vi "API test.vi"() -> ()   [LabVIEW 2014, in "Simple Sequencer TBM tests.lvlib"]
uses:
  Simple Sequencer TBM tests.lvlib
  module/configuration/Simple Sequencer TBM configuration.lvclass
  sequencer parent classes/action configuration parent/action configuration.lvclass
  module/configuration/sequence definition.ctl
  <vilib>/NI/TBM Modules/Sequencer/actions/dwell/Dwell Config.lvclass
  <vilib>/NI/TBM Modules/Sequencer/actions/template action/configuration/Template Action Config.lvclass
  module/execution/Simple Sequencer TBM runtime.lvclass
  simple sequencer api/Simple Sequencer API.lvclass
  <vilib>/NI/TBM Modules/Sequencer/actions/dwell/runtime/Dwell.lvclass
  <vilib>/NI/TBM Modules/Sequencer/actions/template action/runtime/Template Action.lvclass
panel:
  out "String":string
  in  "continue location":i32=-1
  in  "sequences":string[](array[string])
  out "error out 2":errorcluster
  out "error out":errorcluster
  out "available sequences":string[](array[string])
  in  "Resume":bool
  in  "Stop Sequence":bool
  in  "Pause Button":bool
  in  "Play Button":bool
  in  "stop":bool
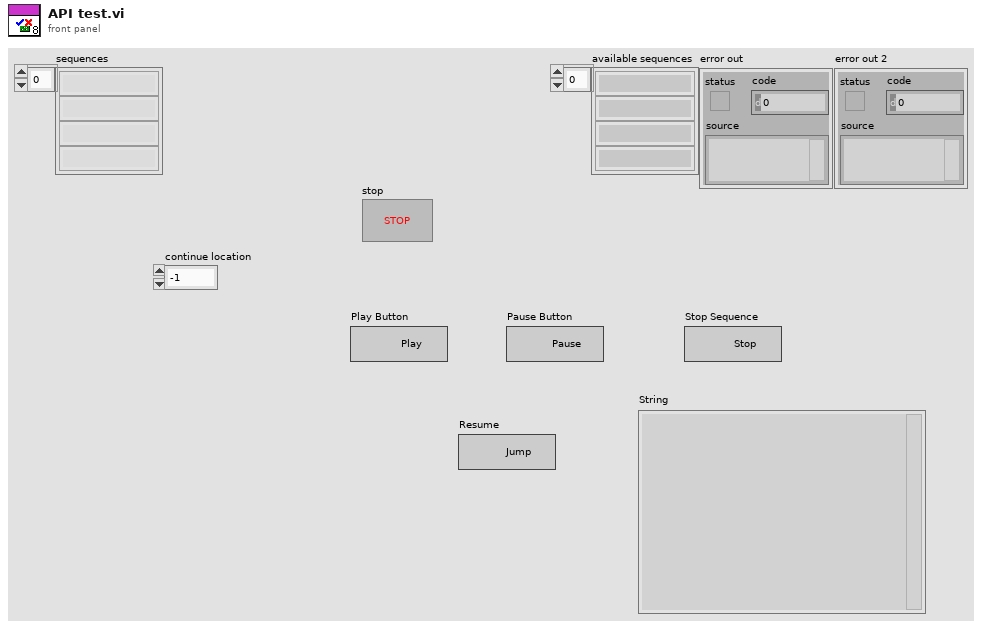
[diagram p1: front panel]
types:
  T1 = typedef "Simple Sequencer TBM configuration.lvclass/sequence definition.ctl" = cluster{"sequence name":string, "action configs":refnum<class "action configuration.lvclass">[]}
  T2 = typedef "TBM channel.lvclass/data tables.ctl" = cluster{"input data":T3, "processing parameter":T3, "processing result":T3, "output data":T3}
  T3 = typedef "tag bus.lvlib/dictionary table pair.ctl" = cluster{"data dictionary":refnum<class "data dictionary.lvclass">, "data table":T4}
  T4 = typedef "tag bus.lvlib/data table.lvlib/data table.ctl" = cluster{"Double":dbl[], "Single":sgl[], "I64":i64[], "I32":i32[], "I16":i16[], "I8":i8[], "U64":u64[], "U32":u32[], "U16":u16[], "U8":u8[], "Boolean":bool[], "String":string[], "Array of Double":cluster{"DBL Array":dbl[]}[], "Array of Single":cluster{"SGL Array":sgl[]}[], "Array of I64":cluster{"I64 Array":i64[]}[], "Array of I32":cluster{"I32 Array":i32[]}[], "Array of I16":cluster{"I16 Array":i16[]}[], "Array of I8":cluster{"I8 Array":i8[]}[], "Array of U64":cluster{"U64 Array":u64[]}[], "Array of U32":cluster{"U32 Array":u32[]}[], "Array of U16":cluster{"U16 Array":u16[]}[], "Array of U8":cluster{"U8 Array":u8[]}[], "Array of Boolean":cluster{"Boolean Array":bool[]}[], "Array of String":cluster{"String Array":string[]}[]}
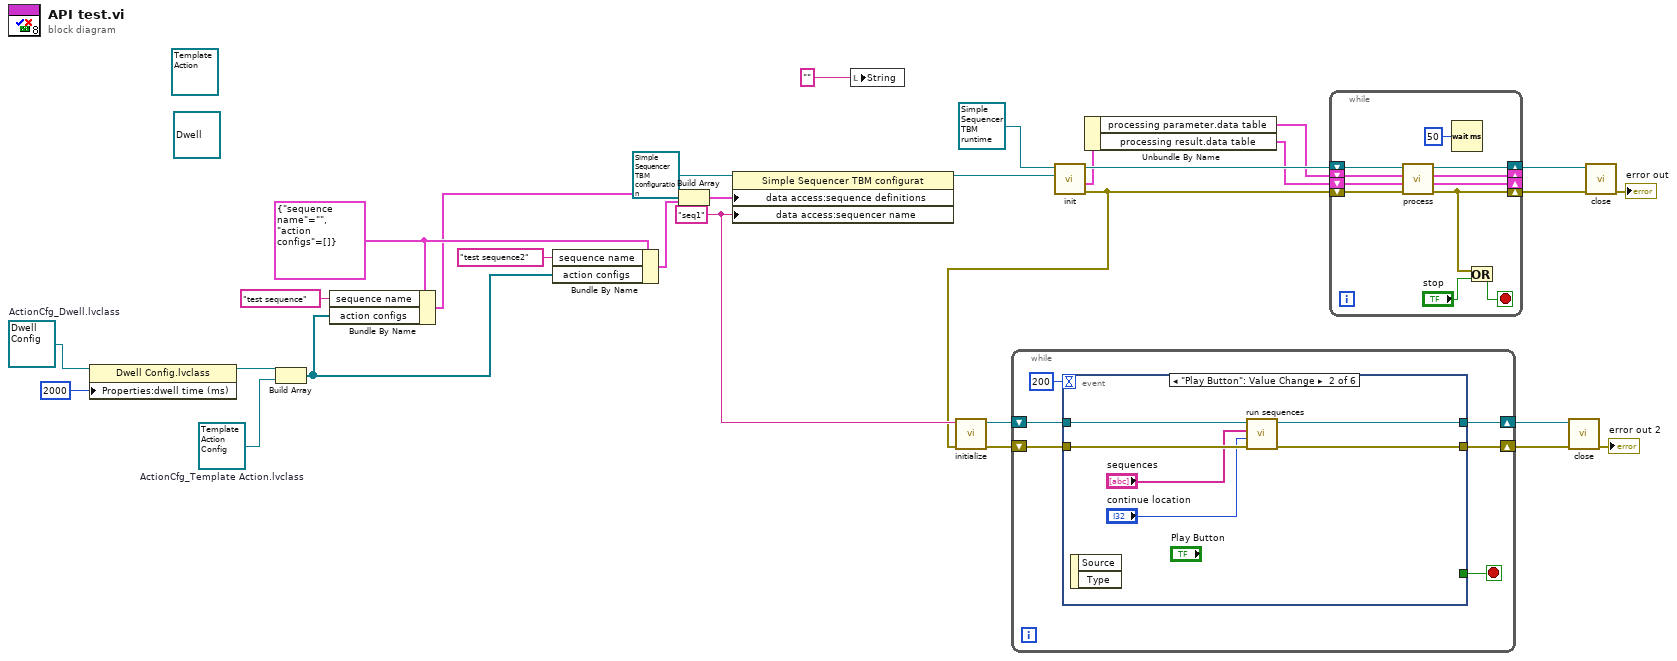
[diagram p0: block diagram]
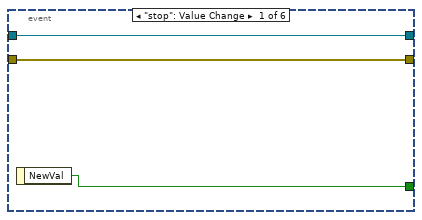
[diagram p2: hidden frame]
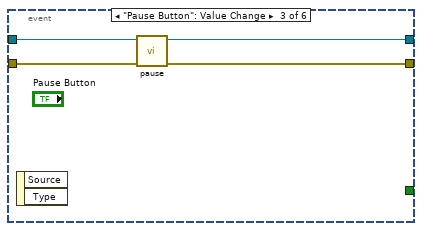
[diagram p3: hidden frame]
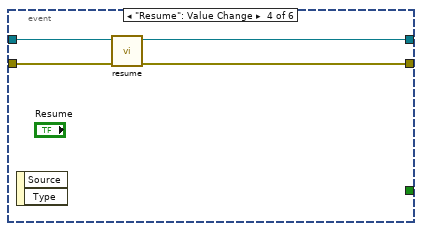
[diagram p4: hidden frame]
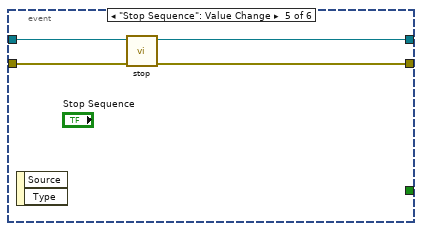
[diagram p5: hidden frame]
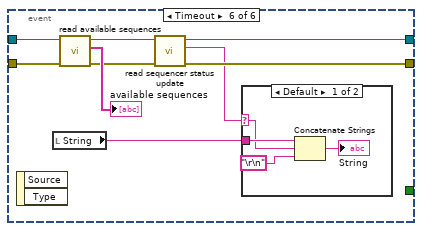
[diagram p6: hidden frame]
diagram:
  (unwired) refnum<class "Template Action.lvclass"> refnum ("Action_Template Action.lvclass")
  (unwired) refnum<class "Dwell.lvclass"> refnum ("Action_Dwell.lvclass")
  w27 = refnum<class "Template Action Config.lvclass"> refnum  # ActionCfg_Template Action.lvclass
  w7 = refnum<class "Dwell Config.lvclass"> refnum  # ActionCfg_Dwell.lvclass
  w25 = T1 {"sequence name"="", "action configs"=[]} ("sequence definitions")
  w15 = "seq1" ("sequencer name")
  n1 = property class="Dwell Config.lvclass"(reference=w7, "Properties:dwell time (ms)"=u32 2000 ("dwell time (ms)")) -> (reference out=w6:refnum<class "Dwell Config.lvclass">)  [unwired: 1 in, 1 out]
  n2 = Build Array(w6, w27) -> (w24:refnum<class>[])
  n3 = Bundle By Name(cluster=w25, "sequence name"="test sequence", "action configs"=w24) -> (w23:T1)
  n4 = Bundle By Name(cluster=w25, "sequence name"="test sequence2", "action configs"=w24) -> (w22:T1)
  n5 = Build Array(w23, w22) -> (w21:T1[])
  n6 = property class="Simple Sequencer TBM configurat"(reference=refnum<class "Simple Sequencer TBM configuration.lvclass"> refnum ("Simple Sequencer TBM configuration"), "data access:sequence definitions"=w21, "data access:sequencer name"=w15) -> (reference out=w20:refnum<class "Simple Sequencer TBM configuration.lvclass">)  [unwired: 1 in, 1 out]
  n7 = local write "String"("" ("String")) -> ()
  n8 = call-dynamic "init.vi"("module configuration"=w20, "Simple Sequencer TBM runtime in"=refnum<class "Simple Sequencer TBM runtime.lvclass"> refnum) -> ("error out"=w3:errorcluster, "data allocations"=w10:T2, "Simple Sequencer TBM runtime out"=w18:refnum<class "Simple Sequencer TBM runtime.lvclass">)  [unwired: 6 in, 1 out]
  n9 = call "initialize.vi"("error in (no error)"=w3, "sequencer name"=w15) -> ("error out"=w13:errorcluster, "Simple Sequencer API out"=w14:refnum<class "Simple Sequencer API.lvclass">)  [unwired: 8 in]
  n10 = while {
    shift-right: [w34] -> w11
    shift-left: w14 -> [w35]
    shift-right: [w31] -> w12
    shift-left: w13 -> [w32]
    stop <- w33 stop-if-true
    n11 = event shown="[1] \"Play Button\": Value Change" {
      selector: _ -> [_ _ _ _ _ _]
      dyn-events: _ -> [_ _ _ _ _ _]
      timeout: 200 -> [_ _ _ _ _ _]
      tunnel: w35 -> [w38 w44 w48 w52 w56 w65]
      tunnel: [w38 w41 w45 w49 w53 w59] -> w34
      tunnel: [w37 _ _ _ _ _] -> w33
      tunnel: w32 -> [w36 w43 w47 w51 w55 w64]
      tunnel: [w36 w42 w46 w50 w54 w60] -> w31
      event "stop": Value Change {
        n12 = event-data() -> ("NewVal"=w37:bool)  [unwired: 1 in]
      }
      event "Play Button": Value Change {
        n13 = event-data() -> ()  [unwired: 1 in, 2 out]
        n14 = call "run sequences.vi"("error in (no error)"=w43, "continue location"="continue location", "sequences"="sequences", "Simple Sequencer API in"=w44) -> ("error out"=w42:errorcluster, "Simple Sequencer API out"=w41:refnum<class "Simple Sequencer API.lvclass">)  [unwired: 6 in]
      }
      event "Pause Button": Value Change {
        n15 = event-data() -> ()  [unwired: 1 in, 2 out]
        n16 = call "pause.vi"("error in (no error)"=w47, "Simple Sequencer API in"=w48) -> ("error out"=w46:errorcluster, "Simple Sequencer API out"=w45:refnum<class "Simple Sequencer API.lvclass">)  [unwired: 8 in]
      }
      event "Resume": Value Change {
        n17 = event-data() -> ()  [unwired: 1 in, 2 out]
        n18 = call "resume.vi"("error in (no error)"=w51, "Simple Sequencer API in"=w52) -> ("error out"=w50:errorcluster, "Simple Sequencer API out"=w49:refnum<class "Simple Sequencer API.lvclass">)  [unwired: 8 in]
      }
      event "Stop Sequence": Value Change {
        n19 = event-data() -> ()  [unwired: 1 in, 2 out]
        n20 = call "stop.vi"("error in (no error)"=w55, "Simple Sequencer API in"=w56) -> ("error out"=w54:errorcluster, "Simple Sequencer API out"=w53:refnum<class "Simple Sequencer API.lvclass">)  [unwired: 8 in]
      }
      event Timeout {
        n21 = event-data() -> ()  [unwired: 1 in, 2 out]
        n22 = local read "String"() -> (w57:string)
        n23 = call "read available sequences.vi"("error in (no error)"=w64, "Simple Sequencer API in"=w65) -> ("error out"=w61:errorcluster, "available sequences"=→"available sequences":string[], "Simple Sequencer API out"=w62:refnum<class "Simple Sequencer API.lvclass">)  [unwired: 7 in]
        n24 = call "read sequencer status update.vi"("error in (no error)"=w61, "Simple Sequencer API in"=w62) -> ("error out"=w60:errorcluster, "Status String"=w58:string, "Simple Sequencer API out"=w59:refnum<class "Simple Sequencer API.lvclass">)  [unwired: 5 in, 2 out]
        n25 = case shown="Default" w58 {
          selector: w58 -> [w67 _]
          tunnel: w57 -> [w69 _]
          frame Default {
            n26 = Concatenate Strings(w69, w67, "\r\n") -> (→"String":string)
          }
          frame "" {
          }
        }
      }
    }
  }
  n27 = Unbundle By Name(w10) -> ("processing parameter.data table"=w9:T4, "processing result.data table"=w8:T4)
  n28 = while {
    shift-right: [w79] -> w17
    shift-left: w18 -> [w80]
    shift-right: [w71] -> w16
    shift-left: w3 -> [w78]
    shift-right: [w76] -> _
    shift-left: w9 -> [w75]
    shift-right: [w73] -> _
    shift-left: w8 -> [w74]
    stop <- w70 stop-if-true
    n29 = call-dynamic "process.vi"("error in"=w78, "result allocation"=w74, "parameters"=w75, "Simple Sequencer TBM runtime in"=w80) -> ("error out"=w71:errorcluster, "results"=w73:T4, "parameter allocation"=w76:T4, "Simple Sequencer TBM runtime out"=w79:refnum<class "Simple Sequencer TBM runtime.lvclass">)  [unwired: 4 in]
    n30 = Wait (ms)(milliseconds to wait=u32 50) -> ()  [unwired: 1 out]
    n31 = Or(x=w71, y="stop") -> (x .or. y?=w70:bool)
  }
  n32 = call "close.vi"("error in (no error)"=w12, "Simple Sequencer API in"=w11) -> ("error out"=→"error out 2":errorcluster)  [unwired: 8 in, 1 out]
  n33 = call-dynamic "close.vi"("error in"=w16, "Simple Sequencer TBM runtime in"=w17) -> ("error out"=→"error out":errorcluster)  [unwired: 9 in]
